vi "TEST INTAKE-SHOOTER.vi"() -> ()   [LabVIEW 2023]
uses:
  ctrl defs/ctrl swerve motor.ctl
  ctrl defs/ctrl MOTOR SELECT.ctl
  <vilib>/Rock Robotics/WPI/ThirdParty/REV Robotics/REVLib/Typedef/Spark MAX Idle Mode.ctl
  ctrl defs/ctrl Spark MAX current limiting.ctl
  ctrl defs/ctrl motor PIDF coefficients.ctl
  <vilib>/Rock Robotics/WPI/ThirdParty/REV Robotics/REVLib/Typedef/Spark MAX Smart Motion Parameters.ctl
  <vilib>/Rock Robotics/WPI/ThirdParty/REV Robotics/REVLib/Typedef/Spark MAX Control Type.ctl
  Global INIT.vi
panel:
  in  "INTAKE speed":dbl(slide) min=-1.0 max=1.0 step=0.01 scale=-1.0..1.0
  in  "LOADER speed":dbl(slide) min=-1.0 max=1.0 step=0.01 scale=-1.0..1.0
  in  "SHOOTER speed":dbl(slide) min=-1.0 max=1.0 step=0.01 scale=-1.0..1.0
  in  "stop":bool
  out "INTAKE motor":T1={"description"="INTAKE", "MOTOR SELECT"=11000, "Installed?"=FALSE, "CAN ID"=11, "refnum name"="ref INTAKE", "Invert"=FALSE, "Idle Mode"=enum."Coast", "Current limiting"={"Linearized"=FALSE, "Free Speed (A)"=20.0, "Primay (A)"=60.0, "Limit RPM (0)"=0}, "MOTOR PIDF coefficients"={"PIDF"={"P Gain"=0.001, "I Gain"=0.0, "D Gain"=0.0, "F Gain"=0.0012, "I Zone"=0.0, "Min Output"=-1.0, "Max Output"=1.0}, "Smart Motion"={"Max Velocity"=1900.0, "Max Acceleration"=750.0, "Minimum Velocity Output"=0.1, "Allowed Closed Loop Error"=0.02}}, "gear ratio"=0.0} {"gear ratio" format="%_5f"; "MOTOR SELECT" items=["REV NEO"=5676, "REV NEO 550"=11000, "VEX Falcon"=6380, "WC Kraken"=6000]}
  out "LOADING motors":T1[](array[typedef])=[{"description"="LOADING CW MOTOR", "MOTOR SELECT"=5676, "Installed?"=FALSE, "CAN ID"=12, "refnum name"="ref LOADER follow", "Invert"=TRUE, "Idle Mode"=enum."Brake", "Current limiting"={"Linearized"=FALSE, "Free Speed (A)"=20.0, "Primay (A)"=60.0, "Limit RPM (0)"=0}, "MOTOR PIDF coefficients"={"PIDF"={"P Gain"=0.001, "I Gain"=0.0, "D Gain"=0.0, "F Gain"=0.0012, "I Zone"=0.0, "Min Output"=-1.0, "Max Output"=1.0}, "Smart Motion"={"Max Velocity"=1900.0, "Max Acceleration"=750.0, "Minimum Velocity Output"=0.1, "Allowed Closed Loop Error"=0.02}}, "gear ratio"=0.0}, {"description"="LOADING CCW MOTOR", "MOTOR SELECT"=5676, "Installed?"=FALSE, "CAN ID"=15, "refnum name"="ref LOADERS", "Invert"=FALSE, "Idle Mode"=enum."Brake", "Current limiting"={"Linearized"=FALSE, "Free Speed (A)"=20.0, "Primay (A)"=60.0, "Limit RPM (0)"=0}, "MOTOR PIDF coefficients"={"PIDF"={"P Gain"=0.001, "I Gain"=0.0, "D Gain"=0.0, "F Gain"=0.0012, "I Zone"=0.0, "Min Output"=-1.0, "Max Output"=1.0}, "Smart Motion"={"Max Velocity"=1900.0, "Max Acceleration"=750.0, "Minimum Velocity Output"=0.1, "Allowed Closed Loop Error"=0.02}}, "gear ratio"=0.0}] {"gear ratio" format="%_5f"; "MOTOR SELECT" items=["REV NEO"=5676, "REV NEO 550"=11000, "VEX Falcon"=6380, "WC Kraken"=6000]}
  out "SHOOTING motors":T1[](array[typedef])=[{"description"="SHOOTER CW MOTOR", "MOTOR SELECT"=11000, "Installed?"=FALSE, "CAN ID"=12, "refnum name"="ref SHOOTER follow", "Invert"=TRUE, "Idle Mode"=enum."Brake", "Current limiting"={"Linearized"=FALSE, "Free Speed (A)"=20.0, "Primay (A)"=60.0, "Limit RPM (0)"=0}, "MOTOR PIDF coefficients"={"PIDF"={"P Gain"=0.001, "I Gain"=0.0, "D Gain"=0.0, "F Gain"=0.0012, "I Zone"=0.0, "Min Output"=-1.0, "Max Output"=1.0}, "Smart Motion"={"Max Velocity"=1900.0, "Max Acceleration"=750.0, "Minimum Velocity Output"=0.1, "Allowed Closed Loop Error"=0.02}}, "gear ratio"=0.0}, {"description"="SHOOTER CCW MOTOR", "MOTOR SELECT"=11000, "Installed?"=FALSE, "CAN ID"=13, "refnum name"="ref SHOOTER", "Invert"=FALSE, "Idle Mode"=enum."Brake", "Current limiting"={"Linearized"=FALSE, "Free Speed (A)"=20.0, "Primay (A)"=60.0, "Limit RPM (0)"=0}, "MOTOR PIDF coefficients"={"PIDF"={"P Gain"=0.001, "I Gain"=0.0, "D Gain"=0.0, "F Gain"=0.0012, "I Zone"=0.0, "Min Output"=-1.0, "Max Output"=1.0}, "Smart Motion"={"Max Velocity"=1900.0, "Max Acceleration"=750.0, "Minimum Velocity Output"=0.1, "Allowed Closed Loop Error"=0.02}}, "gear ratio"=0.0}] {"gear ratio" format="%_5f"; "MOTOR SELECT" items=["REV NEO"=5676, "REV NEO 550"=11000, "VEX Falcon"=6380, "WC Kraken"=6000]}
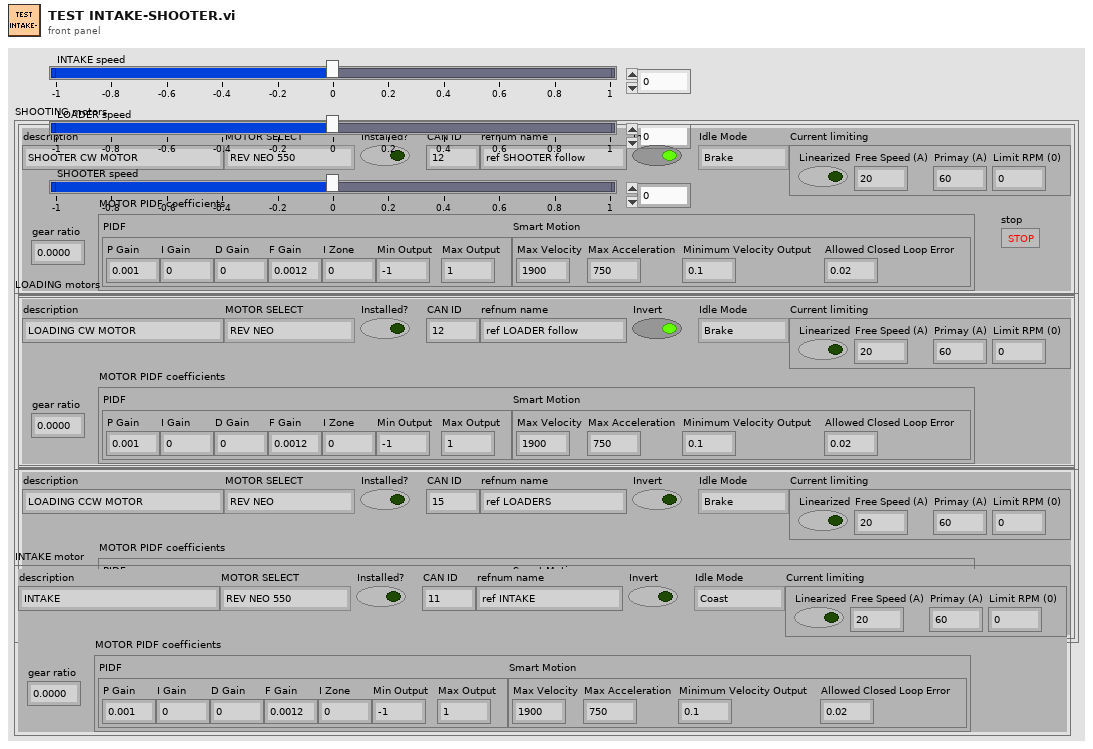
[diagram p1: front panel]
types:
  T1 = typedef "ctrl swerve motor.ctl" = cluster{"description":string, "MOTOR SELECT":T2, "Installed?":bool, "CAN ID":u8, "refnum name":string, "Invert":bool, "Idle Mode":T3, "Current limiting":T4, "MOTOR PIDF coefficients":T5, "gear ratio":dbl}
  T2 = typedef "ctrl MOTOR SELECT.ctl" = i16
  T3 = typedef "Spark MAX Idle Mode.ctl" = enum16{"Coast", "Brake"}
  T4 = typedef "ctrl Spark MAX current limiting.ctl" = cluster{"Linearized":bool, "Free Speed (A)":dbl, "Primay (A)":dbl, "Limit RPM (0)":u32}
  T5 = typedef "ctrl motor PIDF coefficients.ctl" = cluster{"PIDF":cluster{"P Gain":dbl, "I Gain":dbl, "D Gain":dbl, "F Gain":dbl, "I Zone":dbl, "Min Output":dbl, "Max Output":dbl}, "Smart Motion":T6}
  T6 = typedef "Spark MAX Smart Motion Parameters.ctl" = cluster{"Max Velocity":dbl, "Max Acceleration":dbl, "Minimum Velocity Output":dbl, "Allowed Closed Loop Error":dbl}
  T7 = typedef "WPI_MotorControlDeviceRef.ctl" = cluster{"DeviceStatus":errorcluster, "Type":T8, "PWM":cluster{"PWM Channel":T9, "DeadBand":T10}, "CAN":cluster{"Device Number":u8, "SetOutput VI Ref":variant, "GetOutput VI Ref":variant, "Enable VI Ref":variant, "Disable VI Ref":variant, "Data":variant}, "Invert":bool, "DIO PWM":cluster{"PWM \"Enable\" Channel":T9, "DIOChannel":T11, "PWM Rate":dbl}}
  T8 = typedef "WPI_MotorControlType.ctl" = enum16{"PWM", "CAN", "DIO PWM"}
  T9 = typedef "FPGA_DIOPWMChannel.ctl" = enum8{"PWM 0", "PWM 1", "PWM 2", "PWM 3", "PWM 4", "PWM 5", "PWM 6", "PWM 7", "PWM 8", "PWM 9", "PWM MXP 0", "PWM MXP 1", "PWM MXP 2", "PWM MXP 3", "PWM MXP 4", "PWM MXP 5", "PWM MXP 6", "PWM MXP 7", "PWM MXP 8", "PWM MXP 9", "Invalid"}
  T10 = typedef "WPI_PWMDeadband.ctl" = cluster{"Name":string, "maxPositivePwm":i32, "minPositivePwm":i32, "centerPwm":i32, "maxNegativePwm":i32, "minNegativePwm":i32, "angularRange":u16}
  T11 = typedef "FPGA_DIOChannel.ctl" = enum8{"DIO 0", "DIO 1", "DIO 2", "DIO 3", "DIO 4", "DIO 5", "DIO 6", "DIO 7", "DIO 8", "DIO 9", "DIO MXP 0", "DIO MXP 1", "DIO MXP 2", "DIO MXP 3", "DIO MXP 4", "DIO MXP 5", "DIO MXP 6", "DIO MXP 7", "DIO MXP 8", "DIO MXP 9", "DIO MXP 10", "DIO MXP 11", "DIO MXP 12", "DIO MXP 13", "DIO MXP 14", "DIO MXP 15", "SPI Port CS1", "SPI Port CS2", "SPI Port CS3", "SPI Port MISO", "SPI Port MOSI", "Invalid"}
  T12 = typedef "Spark MAX Control Type.ctl" = enum16{"Percent VBus", "Voltage", "Velocity", "Position", "Smart Motion", "Current", "Smart Velocity"}
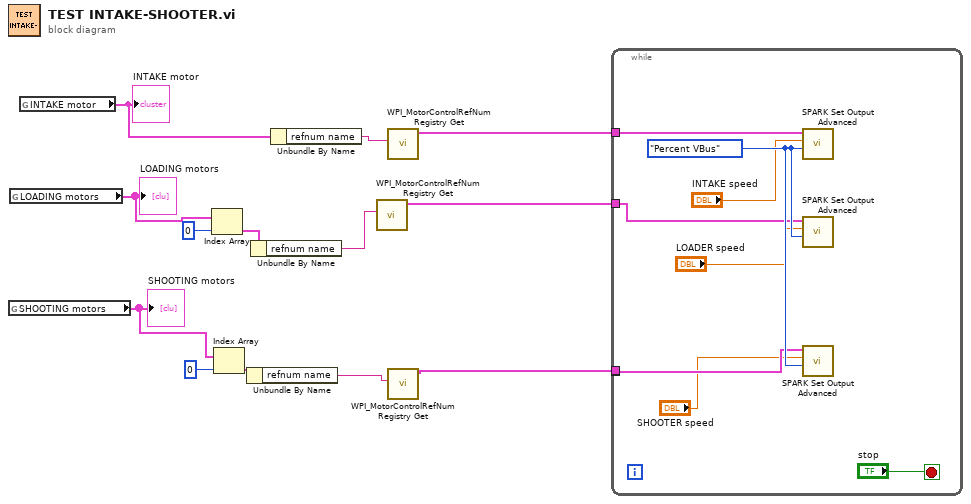
[diagram p0: block diagram]
diagram:
  n1 = global read "Global INIT.vi" "SHOOTING motors"() -> (w8:T1[])
  "SHOOTING motors" <- w8
  n2 = global read "Global INIT.vi" "LOADING motors"() -> (w11:T1[])
  "LOADING motors" <- w11
  n3 = global read "Global INIT.vi" "INTAKE motor"() -> (w13:T1)
  "INTAKE motor" <- w13
  n4 = Index Array(array=w11, index=0) -> (element=w5:T1)
  n5 = Index Array(array=w8, index=0) -> (element=w7:T1)
  n6 = Unbundle By Name(w7) -> ("refnum name"=w6:string)
  n7 = Unbundle By Name(w5) -> ("refnum name"=w4:string)
  n8 = Unbundle By Name(w13) -> ("refnum name"=w12:string)
  n9 = call <vilib>:"WPI_MotorControlRefNum Registry Get.vi"("refnum name"=w4) -> ("MotorControlDevRef"=w2:T7)  [unwired: 9 in, 1 out]
  n10 = call <vilib>:"WPI_MotorControlRefNum Registry Get.vi"("refnum name"=w12) -> ("MotorControlDevRef"=w3:T7)  [unwired: 9 in, 1 out]
  n11 = call <vilib>:"WPI_MotorControlRefNum Registry Get.vi"("refnum name"=w6) -> ("MotorControlDevRef"=w1:T7)  [unwired: 9 in, 1 out]
  n12 = while {
    tunnel: w3 -> [w18]
    tunnel: w2 -> [w19]
    tunnel: [w17] -> _
    tunnel: w1 -> [w17]
    stop <- "stop" stop-if-true
    w20 = Spark_MAX_Control_Type."Percent VBus" ("Control Mode")
    n13 = call <vilib>:"SPARK Set Output Advanced.vi"("Control Mode"=w20, "Setpoint"="INTAKE speed", "MotorControlDevRef"=w18) -> ()  [unwired: 7 in, 2 out]
    n14 = call <vilib>:"SPARK Set Output Advanced.vi"("Control Mode"=w20, "Setpoint"="LOADER speed", "MotorControlDevRef"=w19) -> ()  [unwired: 7 in, 2 out]
    n15 = call <vilib>:"SPARK Set Output Advanced.vi"("Control Mode"=w20, "Setpoint"="SHOOTER speed", "MotorControlDevRef"=w17) -> ()  [unwired: 7 in, 2 out]
  }
